vi "niDTS BT BDR Rx Test Set Parameters.vi"(0 "RX Test Handle In":T8, 7 "BT BDR Parameters":T1={"Channel"=3, "Tx Power (dBm) "=0.0, "External Attenuation (dB)"=0.0, "BDR Packet type"=enum."DH1", "Payload Data"=enum."PN9", "Carrier Mode"=enum."Burst", "Number of Packets"=1500, "Report Period (ms)"=1000.0, "BD ADDRESS"="", "Packet Header"={"LT Address"=0, "Flow"=0, "ARQN"=enum."NAK", "Sequence Bit"=0}, "Dirty Packets"=FALSE, "Corrupt Alternate CRC"=FALSE, "Payload Header"={"LCh"=0, "HeaderFlowControlBit"=FALSE, "Length (-1 AutoSet Max)"=-1}, "Trigger"={"TriggerEdge"=enum."RISing", "TriggerSource"=enum."IMMediate", "TriggerDelay (sec)"=0.0, "TriggerTimeout (sec)"=0.0}}, 11 "error in (no error)":errorcluster) -> (4 "RX Test Handle Out":T8, 15 "error out":errorcluster)   [LabVIEW 2014, in "niDTS BT.lvlib"]
uses:
  niDTS BT.lvlib
  BDR Tx Test/Includes/niDTS BT Rx Test INC Handle.ctl
  Rx Test/Objects/BASE_class/niDTS BT Rx Test.lvclass
  Includes/niDTS BT BDR Rx Test INC Parameters.ctl
  BDR Tx Test/Includes/niDTS BT INC BDR Packet Type.ctl
  Tx Test/Includes/niDTS BT Tx Test INC BD Payload Data.ctl
  Rx Test/Includes/niDTS BT Rx Test INC Carrier Mode.ctl
  Rx Test/Includes/niDTS BT Rx Test INC Packet Header.ctl
  Rx Test/Includes/niDTS BT Rx Test INC Payload Header.ctl
  Includes/niDTS BT DUT INC SG Trigger.ctl
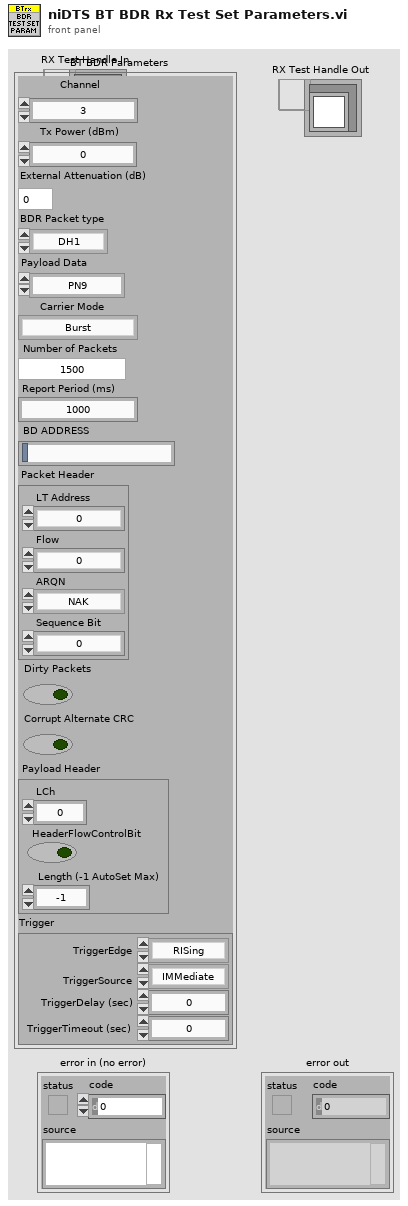
[diagram p1: front panel]
types:
  T1 = typedef "niDTS BT.lvlib/niDTS BT BDR Rx Test INC Parameters.ctl" = cluster{"Channel":i32, "Tx Power (dBm) ":dbl, "External Attenuation (dB)":dbl, "BDR Packet type":T2, "Payload Data":T3, "Carrier Mode":T4, "Number of Packets":i32, "Report Period (ms)":dbl, "BD ADDRESS":string, "Packet Header":T5, "Dirty Packets":bool, "Corrupt Alternate CRC":bool, "Payload Header":T6, "Trigger":T7}
  T2 = typedef "niDTS BT.lvlib/niDTS BT INC BDR Packet Type.ctl" = enum16{"NULL", "POLL", "FHS", "DM1", "DH1", "HV1", "HV2", "HV3", "EV3", "DV", "AUX1", "DM3", "DH3", "EV4", "EV5", "DM5", "DH5"}
  T3 = typedef "niDTS BT.lvlib/niDTS BT Tx Test INC BD Payload Data.ctl" = enum16{"0", "1", "01", "00001111", "PN9", "AUTO"}
  T4 = typedef "niDTS BT.lvlib/niDTS BT Rx Test INC Carrier Mode.ctl" = enum16{"Burst", "Continuous"}
  T5 = typedef "niDTS BT.lvlib/niDTS BT Rx Test INC Packet Header.ctl" = cluster{"LT Address":i8, "Flow":i8, "ARQN":enum16{"NAK", "ACK"}, "Sequence Bit":i8}
  T6 = typedef "niDTS BT.lvlib/niDTS BT Rx Test INC Payload Header.ctl" = cluster{"LCh":i32, "HeaderFlowControlBit":bool, "Length (-1 AutoSet Max)":i32}
  T7 = typedef "niDTS BT.lvlib/niDTS BT DUT INC SG Trigger.ctl" = cluster{"TriggerEdge":enum16{"RISing", "FALLing"}, "TriggerSource":enum16{"IMMediate", "PFI 0", "PFI 1", "RTSI 0", "RTSI 1", "RTSI 2", "RTSI 3", "RTSI 4", "RTSI 5", "RTSI 6", "RTSI 7", "PXI STAR", "Software"}, "TriggerDelay (sec)":dbl, "TriggerTimeout (sec)":dbl}
  T8 = typedef "niDTS BT.lvlib/niDTS BT Rx Test INC Handle.ctl" = refnum<data-value>
  T9 = typedef "niDTS BT.lvlib/niDTS BT Rx Test INC Parameters.ctl" = cluster{"Channel":i32, "Dut Tx Power":dbl, "External Attenuation (dB)":dbl[], "Data Rate":enum16{"1", "2", "3"}, "Packet type":T10, "Payload Data":T3, "Carrier Mode":T4, "Number of Packets":i32, "Report Period (ms)":dbl, "BD ADDRESS":i64, "Dirty Tx":bool, "Corrupt Alternate CRC":bool, "Packet Header":T5, "Payload Header":T6, "Trigger":T7}
  T10 = typedef "niDTS BT.lvlib/niDTS BT INC Packet Type.ctl" = enum16{"NULL", "POLL", "FHS", "DM1", "DH1", "HV1", "HV2", "HV3", "EV3", "DV", "AUX1", "DM3", "DH3", "EV4", "EV5", "DM5", "DH5", "LE-TP"}
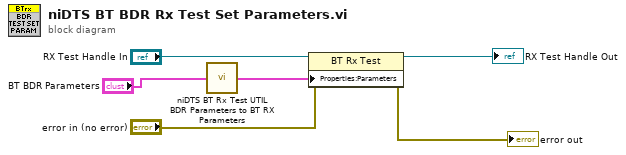
[diagram p0: block diagram]
diagram:
  n1 = call "niDTS BT Rx Test UTIL BDR Parameters to BT RX Parameters.vi"("BT BDR Parameters"="BT BDR Parameters") -> ("BT Rx Parameters"=w2:T9)  [unwired: 14 in]
  n2 = property class="BT Rx Test"(reference="RX Test Handle In", error in="error in (no error)", "Properties:Parameters"=w2) -> (reference out=→"RX Test Handle Out":T8, error out=→"error out":errorcluster)
